vi "ParseJSON.vi"(8 "error in (no error)":errorcluster, 11 "JSON String":string) -> (0 "error out":errorcluster, 3 "BSON Document":refnum<class "tBSONDocument.lvclass">)   [LabVIEW 2013, in "JSON.lvlib" / "tJSONParser.lvclass"]
doc: "Use this VI to parse your JSON document. To parse your JSON document, provide the contents of your JSON string to the JSON String input. Once the parsing is complete, this VI will return a tBSONDocument object that can be queried for elements or serialized into a binary form. See the tBSONDocument documentation for more information."
uses:
  tJSONParser.lvclass
  BSON/tBSONDocument/tBSONDocument.lvclass
  _tokenType.ctl
  tJSONParser.lvclass/tJSONParser.ctl
  _error.ctl
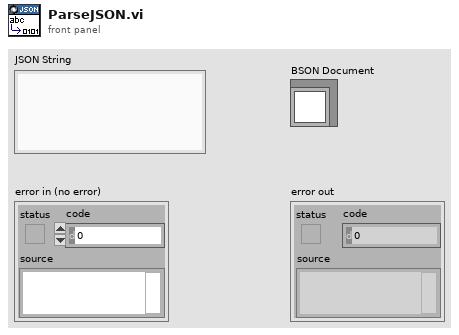
[diagram p1: front panel]
types:
  T1 = typedef "JSON.lvlib/tJSONParser.lvclass/_tokenType.ctl" = enum16{"Object Begin", "Object End", "Array Begin", "Array End", "String Delimeter", "Forward Slash", "Number", "Boolean", "Null", "Object Or Array Separator", "Pair Separator", "End Of File", "Asterisk", "Backward Slash", "Other"}
  T2 = typedef "JSON.lvlib/tJSONParser.lvclass/_error.ctl" = enum16{"Missing Object Open", "Missing Pair Separator", "Missing Object End Or Separator", "Missing Pair String", "Unexpected Token", "Missing Array End Or Separator", "Invalid Escape Sequence", "Unexpected End Of File", "Invalid Unicode", "Unexpected End Of Line", "Invalid Numerical Constant"}
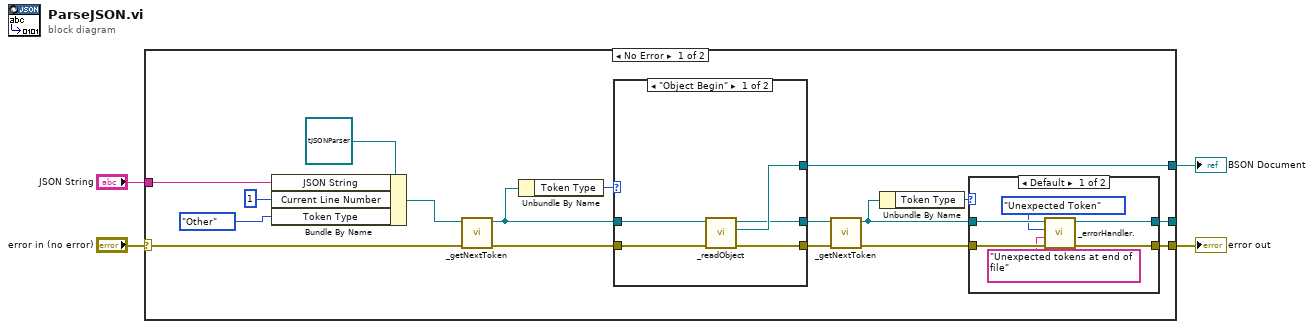
[diagram p0: block diagram]
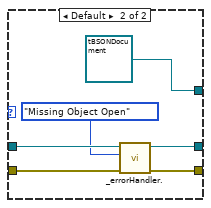
[diagram p3: hidden frame]
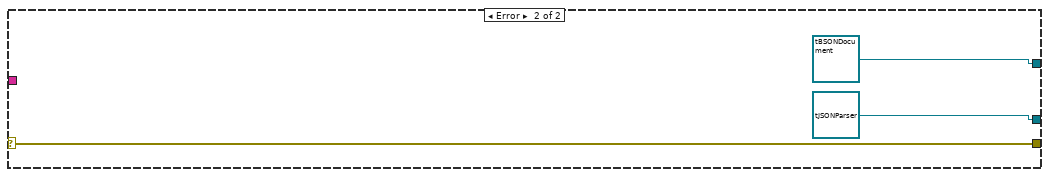
[diagram p4: hidden frame]
diagram:
  n1 = case shown="No Error" "error in (no error)" {
    selector: "error in (no error)" -> [w16 w43]
    tunnel: [w8 w43] -> w3
    tunnel: "JSON String" -> [w20 _]
    tunnel: [w11 refnum<class "tBSONDocument.lvclass"> refnum ("lvMongoDriver.lvlib:BSON.lvlib:tBSONDocument.lvclass")] -> w1
    tunnel: [w6 refnum<class "tJSONParser.lvclass"> refnum ("JSON Parser Out")] -> _
    frame No Error {
      n2 = Bundle By Name(cluster=refnum<class "tJSONParser.lvclass"> refnum ("lvMongoDriver.lvlib:JSON.lvlib:JSONParser.lvclass"), "JSON String"=w20, "Current Line Number"=u32 1, "Token Type"=_tokenType."Other") -> (w17:refnum<class "tJSONParser.lvclass">)
      n3 = call "_getNextToken.vi"("error in (no error)"=w16, "JSON Parser In"=w17) -> ("error out"=w15:errorcluster, "JSON Parser Out"=w14:refnum<class "tJSONParser.lvclass">)  [unwired: 8 in]
      n4 = Unbundle By Name(w14) -> ("Token Type"=w13:T1)
      n5 = case shown="\"Object Begin\"" w13 {
        tunnel: w15 -> [w34 w39]
        tunnel: [w33 w38] -> w12
        tunnel: w14 -> [w32 w37]
        tunnel: [w31 refnum<class "tBSONDocument.lvclass"> refnum ("tBSONDocument out")] -> w11
        tunnel: [w30 w35] -> w10
        frame "Object Begin" {
          n6 = call "_readObject.vi"("error in (no error)"=w34, "JSONParser in"=w32) -> ("error out"=w33:errorcluster, "tBSONDocument out"=w31:refnum<class "tBSONDocument.lvclass">, "JSONParser out"=w30:refnum<class "tJSONParser.lvclass">)  [unwired: 7 in]
        }
        frame Default {
          n7 = call "_errorHandler..vi"("error in (no error)"=w39, "Error Type"=_error."Missing Object Open", "JSON Parser In"=w37) -> ("error out"=w38:errorcluster, "JSON Parser Out"=w35:refnum<class "tJSONParser.lvclass">)  [unwired: 7 in]
        }
      }
      n8 = call "_getNextToken.vi"("error in (no error)"=w12, "JSON Parser In"=w10) -> ("error out"=w7:errorcluster, "JSON Parser Out"=w5:refnum<class "tJSONParser.lvclass">)  [unwired: 8 in]
      n9 = Unbundle By Name(w5) -> ("Token Type"=w9:T1)
      n10 = case shown="Default" w9 {
        tunnel: [w26 w29] -> w8
        tunnel: w7 -> [w27 w29]
        tunnel: [w25 w28] -> w6
        tunnel: w5 -> [w24 w28]
        frame Default {
          n11 = call "_errorHandler..vi"("error in (no error)"=w27, "Additional Text"="Unexpected tokens at end of file", "Error Type"=_error."Unexpected Token", "JSON Parser In"=w24) -> ("error out"=w26:errorcluster, "JSON Parser Out"=w25:refnum<class "tJSONParser.lvclass">)  [unwired: 6 in]
        }
        frame "End Of File" {
        }
      }
    }
    frame Error {
    }
  }
  "BSON Document" <- w1
  "error out" <- w3
